vi "Bind Terminal Value.vi"(4 "Ignore Past Updates? (F)":bool, 6 "Value Changes Only? (T)":bool=TRUE, 7 "Bind by Label (F=Bind by Caption)":bool, 8 "error in (no error)":errorcluster, 9 "Topic Name (Use Control Text)":string, 10 "Ctl Refnum":refnum<vi>, 11 "IObserver in":refnum<class "IObserver.lvclass">) -> (0 "error out":errorcluster, 3 "IObserver out":refnum<class "IObserver.lvclass">)   [LabVIEW 2015, in "IObserver.lvlib" / "IObserver.lvclass"]
doc: "<License>\nCopyright © 2017 Composed Systems, LLC | All rights reserved\nwww.composed.io\n\nAuthor: Ethan Stern <ethan.stern@composed.io>\n\nThis software is provided \"AS IS\" WITHOUT WARRANTIES, either express or implied, AND IS FOR EDUCATIONAL PURPOSES ONLY.\n</License>"
uses:
  IObserver.lvclass
  <vilib>/ActorFramework/Actor/Actor.lvclass/Actor.ctl
  <vilib>/ActorFramework/Message Enqueuer/Message Enqueuer.lvclass/Message Enqueuer.ctl
  IMediator/ISubscriptionPolicy/ISubscriptionPolicy.lvclass
  Mediator/SubscriptionPolicy/ValueChangeSubscription/ValueChangeSubscription.lvclass/ValueChangeSubscription.ctl
  IObserver Messages/Subscribe Msg/Subscribe Msg.lvclass/Subscribe Msg.ctl
  <vilib>/ActorFramework/Message Enqueuer/Init from Existing Queue.vi
  <vilib>/ActorFramework/Message Enqueuer/Enqueue.vi
  <vilib>/ActorFramework/Message Priority Queue/Priority Enqueue.vi
  <vilib>/ActorFramework/Message Enqueuer/Message Enqueuer.lvclass
  Mediator/SubscriptionPolicy/ValueChangeSubscription/ValueChangeSubscription.lvclass
  IObserver Messages/Subscribe Msg/Subscribe Msg.lvclass
  IMediator/SubscriptionRequest/SubscriptionRequest.lvclass
  <vilib>/ActorFramework/Actor/Actor.lvclass
  Mediator/Transport/TerminalBinding/TerminalBinding.lvclass
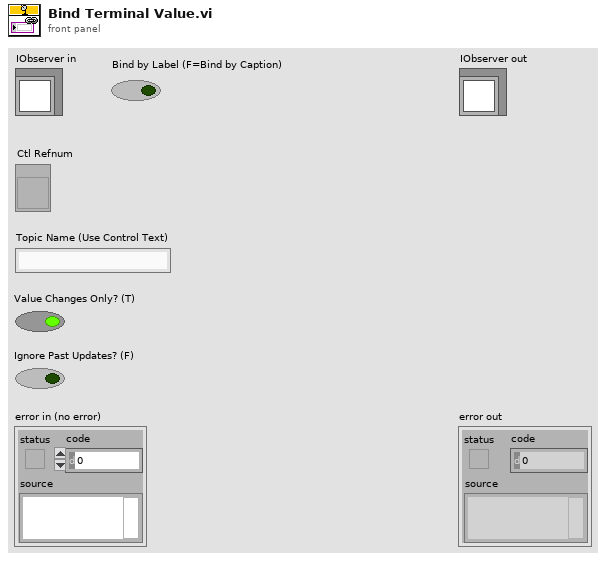
[diagram p1: front panel]
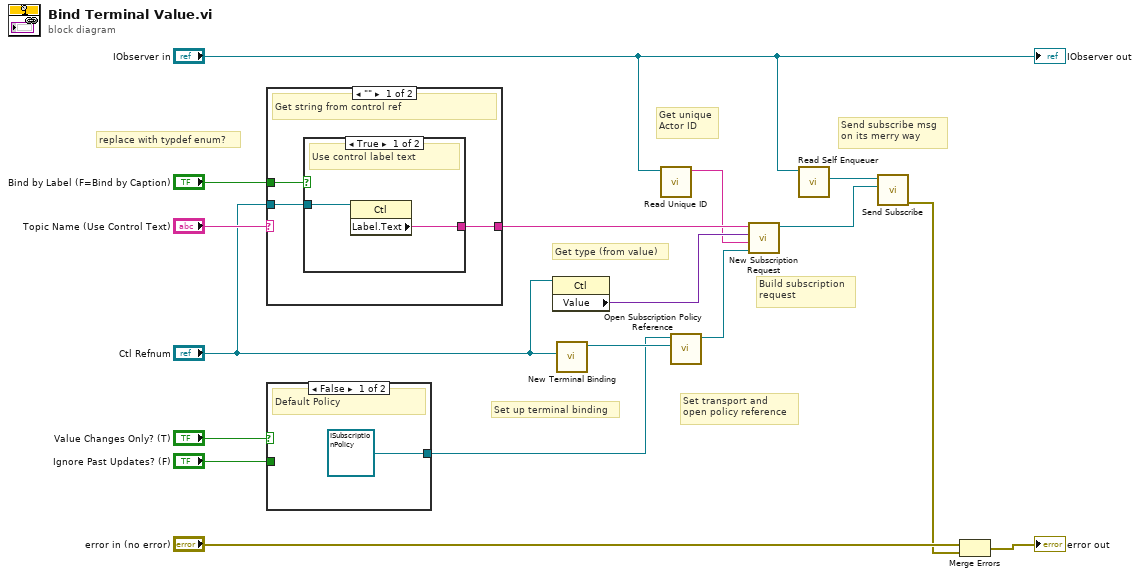
[diagram p0: block diagram]
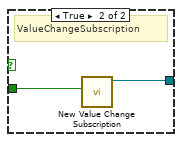
[diagram p2: hidden frame]
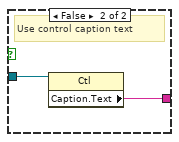
[diagram p3: hidden frame]
diagram:
  # "Set transport and\nopen policy reference"
  # "replace with typdef enum?"
  # "Send subscribe msg\non its merry way"
  # "Build subscription\nrequest"
  # "Get unique\nActor ID"
  # "Get type (from value)"
  # "Set up terminal binding"
  n1 = case shown="\"\"" "Topic Name (Use Control Text)" {
    selector: "Topic Name (Use Control Text)" -> [_ w25]
    tunnel: [w18 w25] -> w8
    tunnel: "Bind by Label (F=Bind by Caption)" -> [w20 _]
    tunnel: "Ctl Refnum" -> [w19 _]
    frame "" {
      # "Get string from control ref"
      n2 = case shown="True" w20 {
        tunnel: w19 -> [w22 w24]
        tunnel: [w21 w23] -> w18
        frame True {
          # "Use control label text"
          n3 = property class="Ctl"(reference=w22) -> ("Label.Text"=w21:string)  [unwired: 1 in, 2 out]
        }
        frame False {
          # "Use control caption text"
          n4 = property class="Ctl"(reference=w24) -> ("Caption.Text"=w23:string)  [unwired: 1 in, 2 out]
        }
      }
    }
    frame Default {
      # "Use string wired to input terminal"
    }
  }
  n5 = case shown="False" "Value Changes Only? (T)" {
    tunnel: "Ignore Past Updates? (F)" -> [_ w28]
    tunnel: [refnum<class "ISubscriptionPolicy.lvclass"> refnum ("IMediator.lvlib:ISubscriptionPolicy.lvclass") w27] -> w2
    frame False {
      # "Default Policy"
    }
    frame True {
      # "ValueChangeSubscription"
      n6 = call "New Value Change Subscription.vi"("Ignore Past Updates? (F)"=w28) -> ("ValueChangeSubscription Out"=w27:refnum<class "ValueChangeSubscription.lvclass">)  [unwired: 10 in]
    }
  }
  n7 = property class="Ctl"(reference="Ctl Refnum") -> ("Value"=w16:variant)  [unwired: 1 in, 2 out]
  n8 = call "New Terminal Binding.vi"("Ctl Refnum"="Ctl Refnum") -> ("TerminalBinding out"=w5:refnum<class "TerminalBinding.lvclass">)  [unwired: 9 in, 1 out]
  n9 = call "Read Unique ID.vi"("IObserver In"="IObserver in") -> ("Unique ID"=w4:string)  [unwired: 10 in]
  n10 = call "Open Subscription Policy Reference.vi"("Transport"=w5, "SubscriptionPolicy"=w2) -> ("Subscription Policy"=w6:refnum<data-value>)  [unwired: 8 in, 1 out]
  n11 = call "New Subscription Request.vi"("Subscription Policy"=w6, "Unique Subscriber ID"=w4, "Type"=w16, "Topic Name"=w8) -> ("SubscriptionRequest"=w13:refnum<class "SubscriptionRequest.lvclass">)  [unwired: 7 in]
  n12 = call <vilib>:"Read Self Enqueuer.vi"("Actor"="IObserver in") -> ("Self Enqueuer"=w14:refnum<class "Message Enqueuer.lvclass">)  [unwired: 10 in]
  n13 = call "Send Subscribe.vi"("SubscriptionRequest"=w13, "Message Enqueuer"=w14) -> ("error out"=w11:errorcluster)  [unwired: 8 in, 1 out]
  n14 = Merge Errors("error in (no error)", w11) -> (→"error out":errorcluster)
  "IObserver out" <- "IObserver in"
